vi "DrawRobot.vi"(8 "Boat (New)":T1, 9 "Boat (Old)":T1, 10 "2D Picture":picture) -> (3 "new picture":picture)   [LabVIEW 2011]
doc: "Draws a magenta circle at the curretn (x,y) coordinates of the Robot in the current mission definition file.\nInputs:\nPicture to draw on\nCluster X\n y coordinates of robot\nOutput:\nmodified picture"
uses:
  WhereAmI.ctl
panel:
  # "Draws a circle at the current x,y coordinates of the robot"
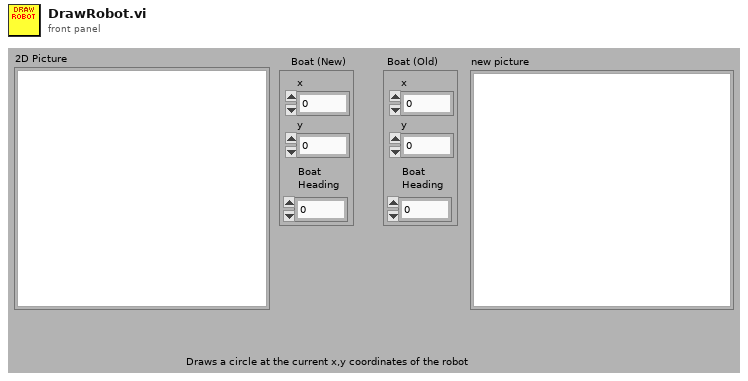
[diagram p1: front panel]
types:
  T1 = typedef "WhereAmI.ctl" = cluster{"x":sgl, "y":sgl, "Boat\nHeading":sgl}
  T2 = cluster{"Width":u16, "Style":enum32{"Solid", "Dash", "Dot", "DashDot", "DashDotDot"}}
  T3 = typedef "imagedata.ctl" = cluster{"image type":i32, "image depth":i32, "image":u8[], "mask":u8[], "colors":u32[], "Rectangle":cluster{"left":i16, "top":i16, "right":i16, "bottom":i16}}
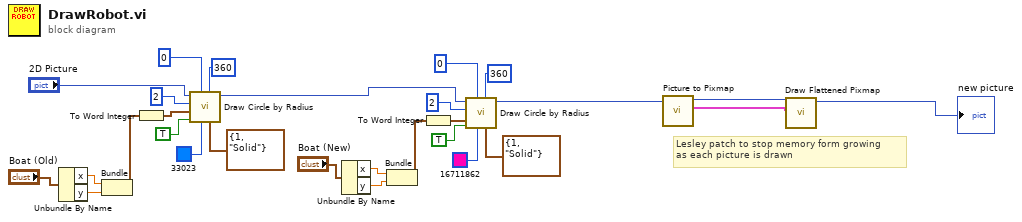
[diagram p0: block diagram]
diagram:
  # "Lesley patch to stop memory form growing\nas each picture is drawn"
  n1 = Unbundle By Name("Boat (Old)") -> ("x"=w13:sgl, "y"=w12:sgl)
  n2 = Bundle("x"=w13, "y"=w12) -> (w11:cluster{"x":sgl, "y":sgl})  [unwired: 1 in]
  n3 = To Word Integer(number=w11) -> (16bit integer=w10:cluster{"x":i16, "y":i16})
  n4 = call <vilib>:"Draw Circle by Radius.vi"("pen"=T2 {"Width"=1, "Style"=enum."Solid"}, "arc size(360)"=i16 360, "color(black)"=u32 33023, "start angle(0)"=i16 0, "fill?(F)"=TRUE, "pixel center"=w10, "radius"=i16 2, "picture"="2D Picture") -> ("new picture"=w15:picture)  [unwired: 3 in]
  n5 = Unbundle By Name("Boat (New)") -> ("x"=w8:sgl, "y"=w7:sgl)
  n6 = Bundle("x"=w8, "y"=w7) -> (w6:cluster{"x":sgl, "y":sgl})  [unwired: 1 in]
  n7 = To Word Integer(number=w6) -> (16bit integer=w5:cluster{"x":i16, "y":i16})
  n8 = call <vilib>:"Draw Circle by Radius.vi"("pen"=T2 {"Width"=1, "Style"=enum."Solid"}, "arc size(360)"=i16 360, "color(black)"=u32 16711862, "start angle(0)"=i16 0, "fill?(F)"=TRUE, "pixel center"=w5, "radius"=i16 2, "picture"=w15) -> ("new picture"=w2:picture)  [unwired: 3 in]
  n9 = call <vilib>:"Picture to Pixmap.vi"("picture"=w2) -> ("image data"=w3:T3, "new picture"=w4:picture)  [unwired: 9 in]
  n10 = call <vilib>:"Draw Flattened Pixmap.vi"("image data"=w3, "picture"=w4) -> ("new picture"=→"new picture":picture)  [unwired: 7 in]
